vi "voltmetr_setup_current_dc.vi"(8 "error in (no error)":errorcluster, 11 "UI in":T1) -> (0 "error out":errorcluster, 3 "UI out":T1)   [LabVIEW 2017]
uses:
  ui.ctl
  classes/dc_power_supply/DC_power_supply.lvclass
  ui_buttons.ctl
  types/boc_type.ctl
  <instrlib>/PICOTEST M352XA/Public/Controls/Function.ctl
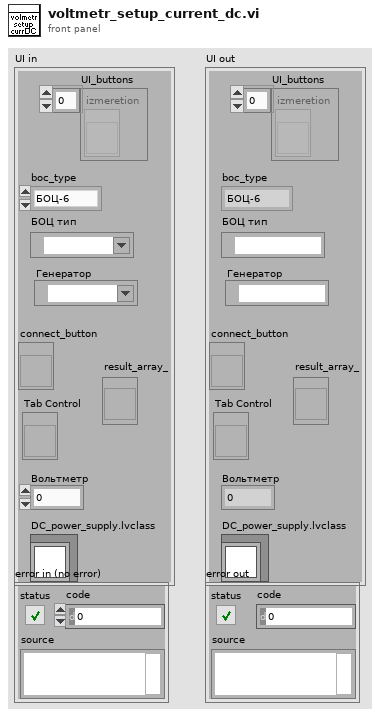
[diagram p1: front panel]
types:
  T1 = typedef "ui.ctl" = cluster{"UI_buttons":T2, "Tab Control":refnum<vi>, "connect_button":refnum<vi>, "generator":refnum<visa-resource-name>, "voltmetr":refnum<visa-resource-name>, "channel_timeout_sec":dbl, "boc_type":T3, "result_array_":refnum<vi>, "DC_power_supply.lvclass":refnum<class "DC_power_supply.lvclass">}
  T2 = typedef "ui_buttons.ctl" = refnum<vi>[]
  T3 = typedef "boc_type.ctl" = enum16{"БОЦ-6", "БОЦ-12"}
  T4 = typedef "Function.ctl" = enum16{"VOLTage:DC", "VOLTage:DC:RATio", "VOLTage:AC", "CURRent:DC", "CURRent:AC", "RESistance", "FRESistance", "FREQuency", "PERiod", "FREQuency:CURRent", "PERiod:CURRent", "CAPacitance", "CONTinuity", "DIODe", "TCOuple", "TEMPerature"}
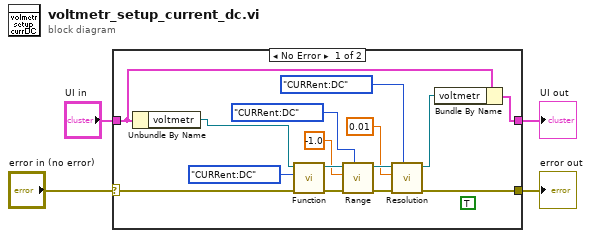
[diagram p0: block diagram]
diagram:
  n1 = case shown="No Error" "error in (no error)" {
    selector: "error in (no error)" -> [w16 w21]
    tunnel: [w19 w20] -> w1
    tunnel: "UI in" -> [w18 w20]
    tunnel: [w9 w21] -> w3
    frame No Error {
      (unwired) TRUE ("Reset (True)")
      n2 = Unbundle By Name(w18) -> ("voltmetr"=w17:refnum<visa-resource-name>)
      n3 = call <instrlib>:"Function.vi"("error in (no error)"=w16, "Function"=Function."CURRent:DC", "VISA resource name"=w17) -> ("error out"=w11:errorcluster, "VISA resource name out"=w14:refnum<visa-resource-name>)  [unwired: 6 in, 1 out]
      n4 = call <instrlib>:"Range.vi"("Function"=Function."CURRent:DC", "error in (no error)"=w11, "Range"=-1.0, "VISA resource name"=w14) -> ("error out"=w10:errorcluster, "VISA resource name out"=w13:refnum<visa-resource-name>)  [unwired: 5 in, 1 out]
      n5 = call <instrlib>:"Resolution.vi"("Function"=Function."CURRent:DC", "error in (no error)"=w10, "Resolution"=0.01, "VISA resource name"=w13) -> ("error out"=w9:errorcluster, "VISA resource name out"=w12:refnum<visa-resource-name>)  [unwired: 5 in, 1 out]
      n6 = Bundle By Name(cluster=w18, "voltmetr"=w12) -> (w19:T1)
    }
    frame Error {
    }
  }
  "UI out" <- w1
  "error out" <- w3
